vi "Real-Time LED-Core_Initialize.vi"(0 "Initialization Sequence":string, 5 "FTW Actor Instance Configuration":string, 11 "error in (no error)":errorcluster) -> (4 "Actor Template-Core out":refnum<class "Real-Time LED-Core.lvclass">, 6 "Incoming Requests":refnum<event-registration>, 8 "Local Messages":refnum<event-registration>, 15 "error out":errorcluster)   [LabVIEW 2013, in "Real-Time LED-Core.lvclass"]
uses:
  Real-Time LED-Core.lvclass
  source/actor/Message/Request/FTW-Message-IncomingRequest.lvclass
  source/actor/Message/Base/FTW-Message.lvclass
  Real-Time LED-Core.lvclass/Real-Time LED-Core.ctl
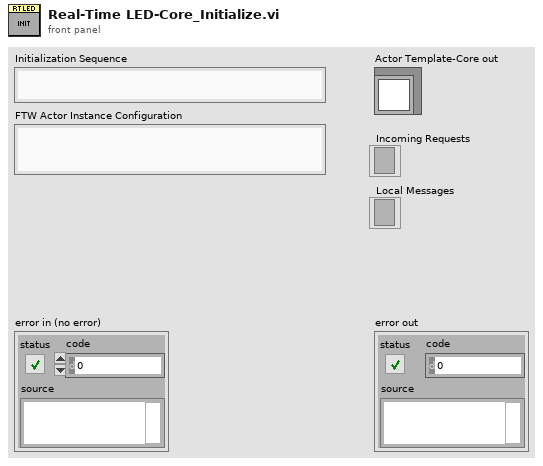
[diagram p1: front panel]
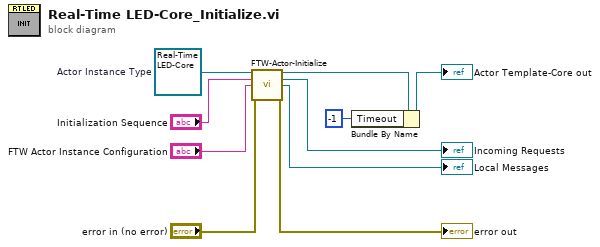
[diagram p0: block diagram]
diagram:
  w10 = refnum<class "Real-Time LED-Core.lvclass"> refnum  # Actor Instance Type
  n1 = call-dynamic "FTW-Actor-Initialize.vi"("FTW Actor Instance Type"=w10, "Initialization Job Sequence"="Initialization Sequence", "Actor Instance Configuration"="FTW Actor Instance Configuration", "error in"="error in (no error)") -> ("FTW Actor Instance"=w9:refnum<class "Real-Time LED-Core.lvclass">, "Incoming Requests"=→"Incoming Requests":refnum<event-registration>, "Local Messages"=→"Local Messages":refnum<event-registration>, "error out"=→"error out":errorcluster)  [unwired: 8 in]
  n2 = Bundle By Name(cluster=w9, "Timeout"=-1) -> (→"Actor Template-Core out":refnum<class "Real-Time LED-Core.lvclass">)
